vi "2eme_ordre_numerique_AhmedAmrani.vi"(4 "RAZ":bool, 6 "e_n":dbl, 7 "T":dbl=0.25, 8 "a2":dbl=1.0, 9 "a1":dbl=1.0, 10 "a0":dbl=1.0, 11 "b0":dbl=1.0) -> (5 "y_n":dbl)   [LabVIEW 2012]
panel:
  out "Waveform Chart":cluster{"y_n":dbl, "e_n":dbl}(graph)={"y_n"=5.992595411754822, "e_n"=1.0}
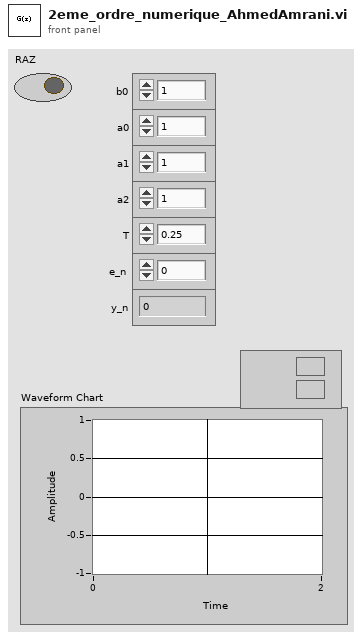
[diagram p1: front panel]
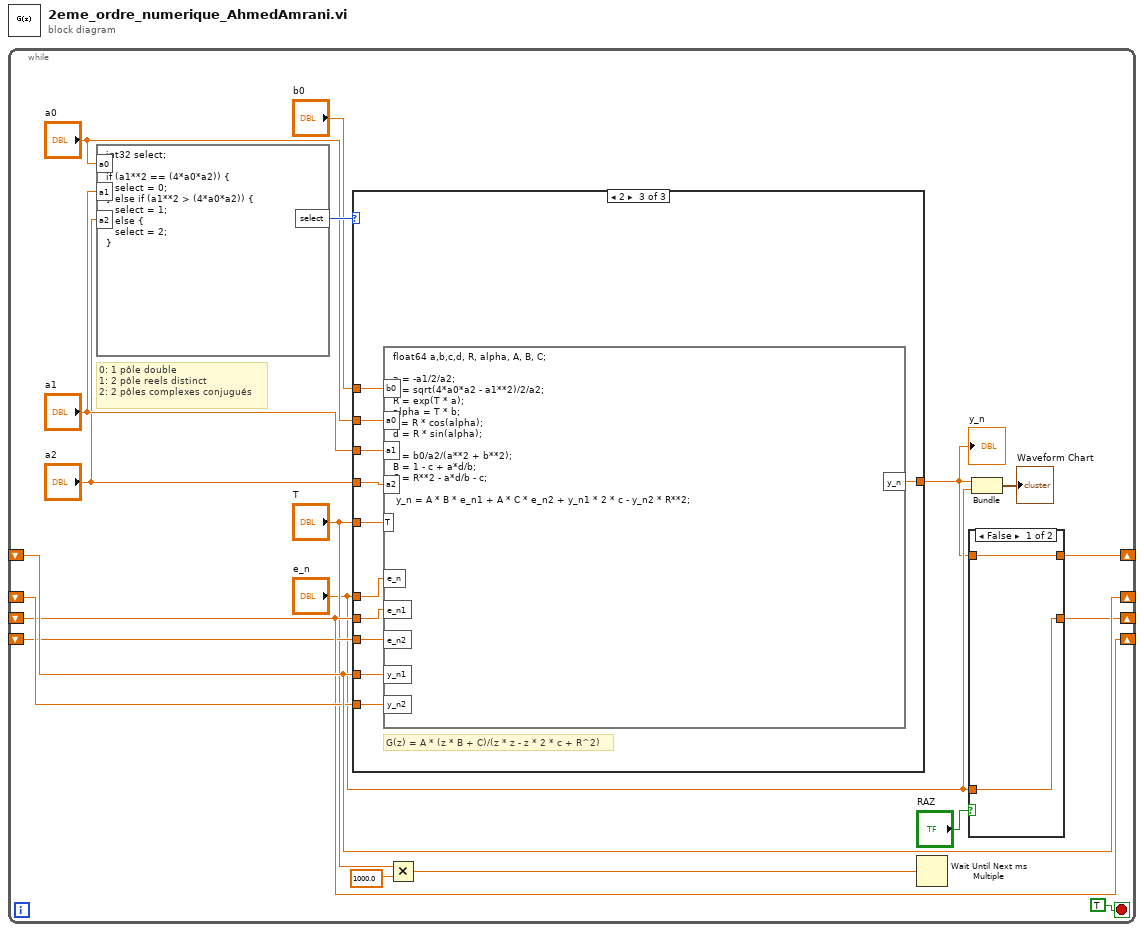
[diagram p0: block diagram]
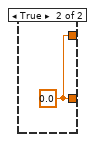
[diagram p2: hidden frame]
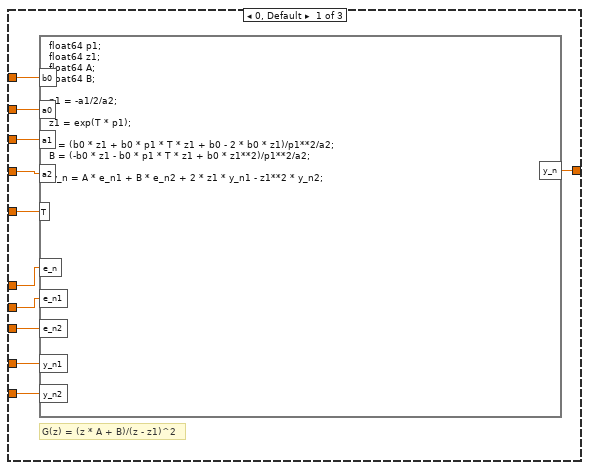
[diagram p3: hidden frame]
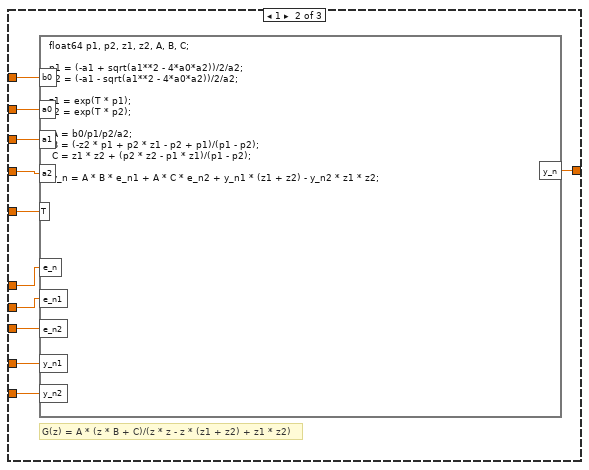
[diagram p4: hidden frame]
diagram:
  n1 = while {
    shift-right: [w1] -> _
    shift-left: _ -> [w19]
    shift-right: [w19] -> _
    shift-left: _ -> [w18]
    shift-right: [w4] -> _
    shift-left: _ -> [w17]
    shift-right: [w17] -> _
    shift-left: _ -> [w16]
    stop <- TRUE stop-if-true
    # "0: 1 pôle double\n1: 2 pôle reels distinct\n2: 2 pôles complexes conjugués"
    n2 = formula code="int32 select;\n\nif (a1**2 == (4*a0*a2)) {\n   select = 0;\n} else if (a1**2 > (4*a0*a2)) {\n   select = 1;\n} else {\n   select = 2;\n}"("a0"="a0", "a1"="a1", "a2"="a2") -> ("select"=w11:i32)
    n3 = case shown="2" w11 {
      tunnel: "b0" -> [w27 w44 w54]
      tunnel: "a0" -> [w28 w43 w53]
      tunnel: "a1" -> [w29 w42 w52]
      tunnel: "a2" -> [w30 w41 w51]
      tunnel: "T" -> [w32 w40 w50]
      tunnel: "e_n" -> [w31 w39 w49]
      tunnel: [w33 w38 w55] -> w2
      tunnel: w19 -> [w26 w37 w46]
      tunnel: w18 -> [w25 w36 w45]
      tunnel: w17 -> [w24 w35 w48]
      tunnel: w16 -> [w23 w34 w47]
      frame 0, Default {
        # "G(z) = (z * A + B)/(z - z1)^2"
        n4 = formula code="float64 p1; \nfloat64 z1;\nfloat64 A;\nfloat64 B;\n\np1 = -a1/2/a2;\n\nz1 = exp(T * p1);\n\nA = (b0 * z1 + b0 * p1 * T * z1 + b0 - 2 * b0 * z1)/p1**2/a2;\nB = (-b0 * z1 - b0 * p1 * T * z1 + b0 * z1**2)/p1**2/a2;\n    \n y_n = A * e_n1 + B * e_n2 + 2 * z1 * y_n1 - z1**2 * y_n2;"("b0"=w27, "a0"=w28, "a1"=w29, "a2"=w30, "T"=w32, "e_n"=w31, "e_n1"=w24, "e_n2"=w23, "y_n1"=w26, "y_n2"=w25) -> ("y_n"=w33:dbl)
      }
      frame 1 {
        # "G(z) = A * (z * B + C)/(z * z - z * (z1 + z2) + z1 * z2)"
        n5 = formula code="float64 p1, p2, z1, z2, A, B, C;\n\np1 = (-a1 + sqrt(a1**2 - 4*a0*a2))/2/a2;\np2 = (-a1 - sqrt(a1**2 - 4*a0*a2))/2/a2;\n\nz1 = exp(T * p1);\nz2 = exp(T * p2);\n\n A = b0/p1/p2/a2;\n B = (-z2 * p1 + p2 * z1 - p2 + p1)/(p1 - p2);\n C = z1 * z2 + (p2 * z2 - p1 * z1)/(p1 - p2);\n\n y_n = A * B * e_n1 + A * C * e_n2 + y_n1 * (z1 + z2) - y_n2 * z1 * z2;"("b0"=w44, "a0"=w43, "a1"=w42, "a2"=w41, "T"=w40, "e_n"=w39, "e_n1"=w35, "e_n2"=w34, "y_n1"=w37, "y_n2"=w36) -> ("y_n"=w38:dbl)
      }
      frame 2 {
        # "G(z) = A * (z * B + C)/(z * z - z * 2 * c + R^2)"
        n6 = formula code="float64 a,b,c,d, R, alpha, A, B, C;\n\na = -a1/2/a2;\nb = sqrt(4*a0*a2 - a1**2)/2/a2;\nR = exp(T * a);\nalpha = T * b;\nc = R * cos(alpha);\nd = R * sin(alpha);\n\nA = b0/a2/(a**2 + b**2);\nB = 1 - c + a*d/b;\nC = R**2 - a*d/b - c;\n\n y_n = A * B * e_n1 + A * C * e_n2 + y_n1 * 2 * c - y_n2 * R**2;"("b0"=w54, "a0"=w53, "a1"=w52, "a2"=w51, "T"=w50, "e_n"=w49, "e_n1"=w48, "e_n2"=w47, "y_n1"=w46, "y_n2"=w45) -> ("y_n"=w55:dbl)
      }
    }
    "y_n" <- w2
    n7 = Multiply(x="T", y=1000.0) -> (x*y=w12:dbl)
    n8 = Wait Until Next ms Multiple(millisecond multiple=w12) -> ()  [unwired: 1 out]
    n9 = case shown="False" "RAZ" {
      tunnel: [w21 w22] -> w4
      tunnel: "e_n" -> [w21 _]
      tunnel: w2 -> [w20 _]
      tunnel: [w20 w22] -> w1
      frame False {
      }
      frame True {
        w22 = 0.0 ("y_n")
      }
    }
    n10 = Bundle("y_n"=w2, "e_n"="e_n") -> (→"Waveform Chart":cluster{"y_n":dbl, "e_n":dbl})  [unwired: 1 in]
  }
